vi "Find All.vi"(9 "Data to Match":variant, 11 "Data":variant[](array[variant])) -> (3 "Indicies":i32[](array[numeric]))   [LabVIEW 2015]
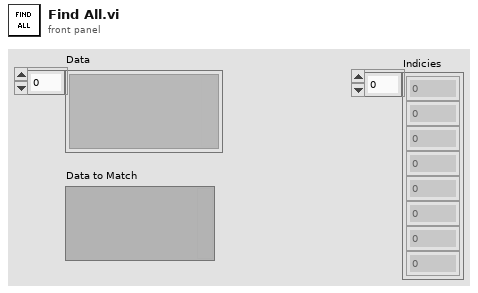
[diagram p1: front panel]
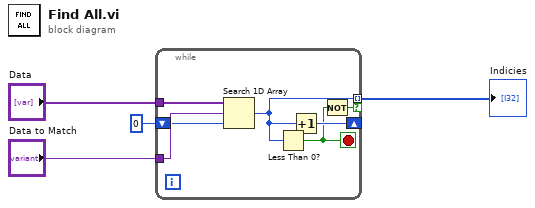
[diagram p0: block diagram]
diagram:
  n1 = while {
    tunnel: "Data" -> [w11]
    tunnel: "Data to Match" -> [w10]
    shift-right: [w7] -> _
    shift-left: 0 -> [w9]
    tunnel: [w8] -> w1 mode=indexing if=w5
    stop <- w6 stop-if-true
    n2 = Search 1D Array(1D array=w11, element=w10, start index (0)=w9) -> (index of element=w8:i32)
    n3 = Less Than 0?(x=w8) -> (x < 0?=w6:bool)
    n4 = Increment(x=w8) -> (x+1=w7:i32)
    n5 = Not(x=w6) -> (.not. x?=w5:bool)
  }
  "Indicies" <- w1
